vi "delete_old_methods.vi"(8 "error in (no error)":errorcluster, 11 "Path":path) -> (0 "error out":errorcluster)   [LabVIEW 2020]
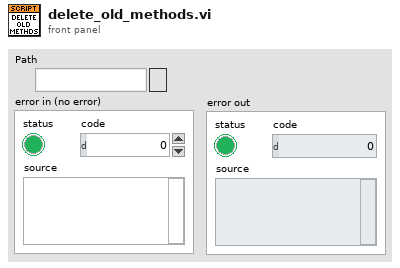
[diagram p1: front panel]
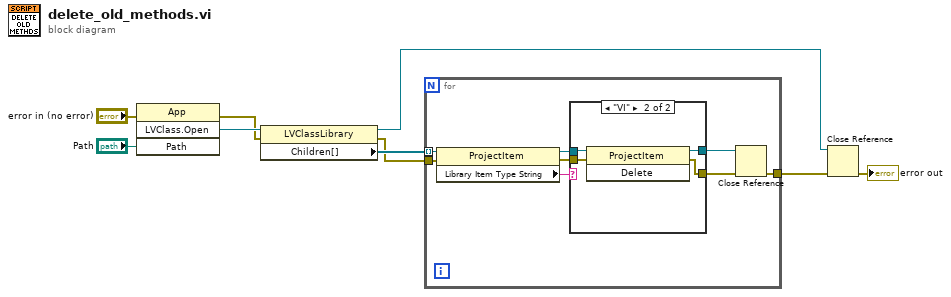
[diagram p0: block diagram]
diagram:
  n1 = invoke class="App" method="LVClass.Open"(error in="error in (no error)", "Path"="Path") -> (error out=w5:errorcluster, "LVClass.Open"=w8:refnum<vi>)  [unwired: 2 in, 2 out]
  n2 = property class="LVClassLibrary"(reference=w8, error in=w5) -> (reference out=w2:refnum<vi>, error out=w6:errorcluster, "Children[]"=w7:refnum<vi>[])
  n3 = for {
    tunnel: w7 -> [w17] mode=indexing
    tunnel: w6 -> [w13]
    tunnel: [w10] -> w3
    n4 = property class="ProjectItem"(reference=w17, error in=w13) -> (reference out=w15:refnum<vi>, error out=w14:errorcluster, "Library Item Type String"=w16:string)
    n5 = case shown="\"VI\"" w16 {
      tunnel: w15 -> [w19 w23]
      tunnel: w14 -> [w18 w22]
      tunnel: [w19 w21] -> w12
      tunnel: [w18 w20] -> w11
      frame "False", Default {
      }
      frame "VI" {
        n6 = invoke class="ProjectItem" method="Delete"(reference=w23, error in=w22) -> (reference out=w21:refnum<vi>, error out=w20:errorcluster)  [unwired: 1 in, 1 out]
      }
    }
    n7 = Close Reference(reference=w12, error in (no error)=w11) -> (error out=w10:errorcluster)
  }
  n8 = Close Reference(reference=w2, error in (no error)=w3) -> (error out=→"error out":errorcluster)
